vi "K2182A_Merge_Cluster.vi"(1 "K2182A Control":T3, 2 "AMI_Status":T4) -> (0 "K2182A Cluster":T1={"Plot Window"=[], "Range"=1.0, "Update"=FALSE, "Range selector"=enum."10mV", "Auto Range"=FALSE, "V"=0.0, "Auto Range set"=FALSE})   [LabVIEW 2019]
uses:
  K2812A/K2812A_status.ctl
  K2812A/K2812A_control.ctl
  Equipment/Keithley 622x/Configure/2182 -A/Low Level/Typedefs/KE2182 -- Voltage Ranges.ctl
  K2812A/K2812A_cluster.ctl
  Equipment/Keithley 622x/Keithley 622x.lvlib
panel:
  # "K 2182A"
  # "K 2182A"
  # "K 2182A"
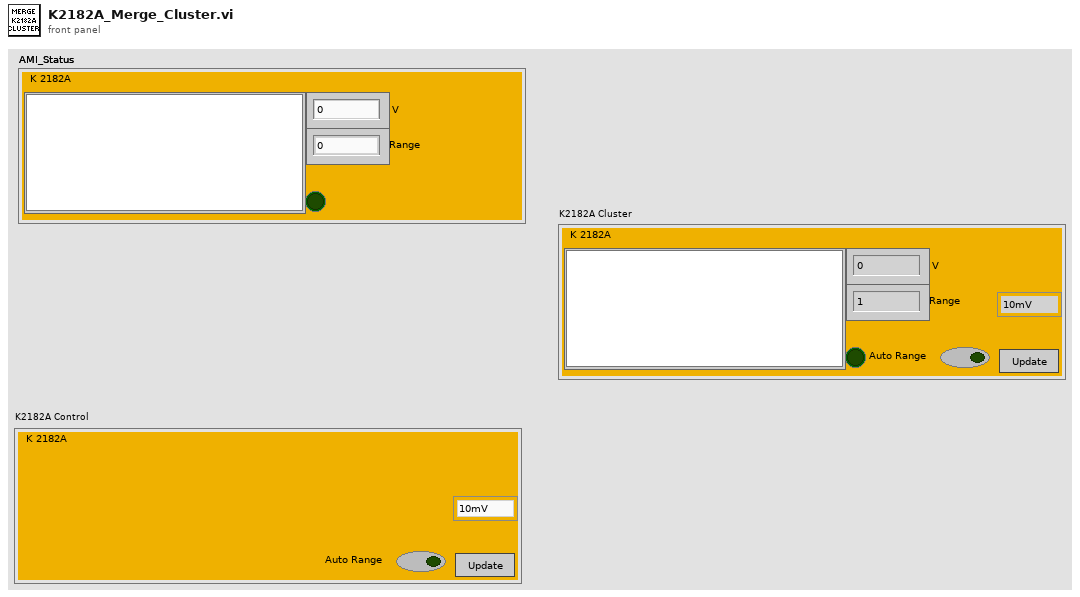
[diagram p1: front panel]
types:
  T1 = typedef "K2812A_cluster.ctl" = cluster{"Plot Window":dbl[][], "Range":dbl, "Update":bool, "Range selector":T2, "Auto Range":bool, "V":dbl, "Auto Range set":bool}
  T2 = typedef "Keithley 622x.lvlib/KE2182 -- Voltage Ranges.ctl" = enum16{"10mV", "100mV", "1V", "10V", "100V"}
  T3 = typedef "K2812A_control.ctl" = cluster{"Update":bool, "Range selector":T2, "Auto Range":bool}
  T4 = typedef "K2812A_status.ctl" = cluster{"Plot Window":dbl[][], "Range":dbl, "V":dbl, "Auto Range set":bool}
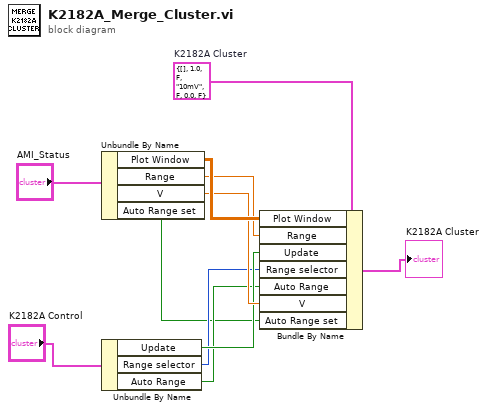
[diagram p0: block diagram]
diagram:
  w11 = T1 {"Plot Window"=[], "Range"=1.0, "Update"=FALSE, "Range selector"=enum."10mV", "Auto Range"=FALSE, "V"=0.0, "Auto Range set"=FALSE}  # K2182A Cluster
  n1 = Unbundle By Name("AMI_Status") -> ("Plot Window"=w7:dbl[][], "Range"=w6:dbl, "V"=w5:dbl, "Auto Range set"=w1:bool)
  n2 = Unbundle By Name("K2182A Control") -> ("Update"=w4:bool, "Range selector"=w3:T2, "Auto Range"=w2:bool)
  n3 = Bundle By Name(cluster=w11, "Plot Window"=w7, "Range"=w6, "Update"=w4, "Range selector"=w3, "Auto Range"=w2, "V"=w5, "Auto Range set"=w1) -> (→"K2182A Cluster":T1)
